vi "Configure-cameras.vi"(7 "Correct. params. ref.":refnum<data-value>, 8 "error in":errorcluster, 10 "Acquis. params. ref.":refnum<data-value>, 11 "Config. params. ref in.":refnum<data-value>) -> (0 "error IO":errorcluster, 3 "Config. params. ref.":refnum<data-value>, 5 "Succes?":bool)   [LabVIEW 2013, in "CameraVision.lvlib" / "CV-Configuration.lvclass"]
uses:
  CV-Configuration.lvclass
  Acquisition/CV-Acquisition.lvclass
  Correction/CV-Correction.lvclass
  Hardware/Camera/PF_MV1-D1312-240/PF_MV1-D1312-240.lvclass
  Hardware/Camera/Camera.lvclass
  UI/Module-states.ctl
  UI/Popup-messages.ctl
  Acquisition/CV-Acquisition.lvclass/CV-Acquisition.ctl
  CV-Configuration.lvclass/CV-Configuration.ctl
  Acquisition/Read Trigger mode.vi
  Acquisition/Read Maximum frame rate.vi
  Read Camport array.vi
  Read Framegrabber board.vi
  Read ROI width.vi
  Read ROI height.vi
  Read X-offsets.vi
  Read Y-offsets.vi
  Write Camera array.vi
  Write Camera status.vi
  UI/CV-UI.lvclass
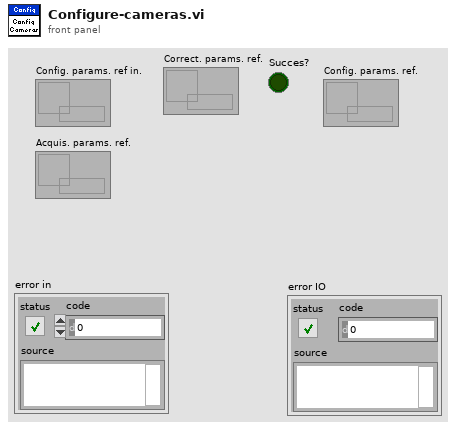
[diagram p1: front panel]
types:
  T1 = typedef "CameraVision.lvlib/CV-UI.lvclass/Popup-messages.ctl" = enum16{"Error-Black image", "Error-Camera config file", "Error-Camera connect", "Error-Grabber init", "Error-Camera setting", "Error-Image offset", "Error-Image import", "Error-Settings file not exist", "Error-Timing source", "Conflict-Filters", "Conflict-Map", "Conflict-Framerate", "Conflict-Charact", "Conflict-Temperature field", "Conflict-Temperature value", "Conflict-Storage-Binary image", "Conflict-Storage-Corrected image", "Conflict-Storage-Map", "Conflict-Storage-Charact", "Conflict-Storage-Temperature field", "Conflict-Storage-Temperature value", "Warning-File exist", "Warning-Parameter reset", "Warning-User cancel", "Info-Images imported"}
  T2 = typedef "CameraVision.lvlib/CV-UI.lvclass/Module-states.ctl" = enum16{"Inactive", "Active", "Data-loss", "Error", "Simulation", "Synchronizing", "Initialized", "Released"}
  T3 = typedef "Trigger-modes.ctl" = enum16{"Camera timed (not sync.)", "Framegrabber timed (sync.)", "Software timed (sync.)", "External timing (sync.)", "Manual (sync.)", "Gated - camera (not sync.)", "Gated - grabber (sync.)", "Gated - software (sync.)", "Gated - external (sync.)"}
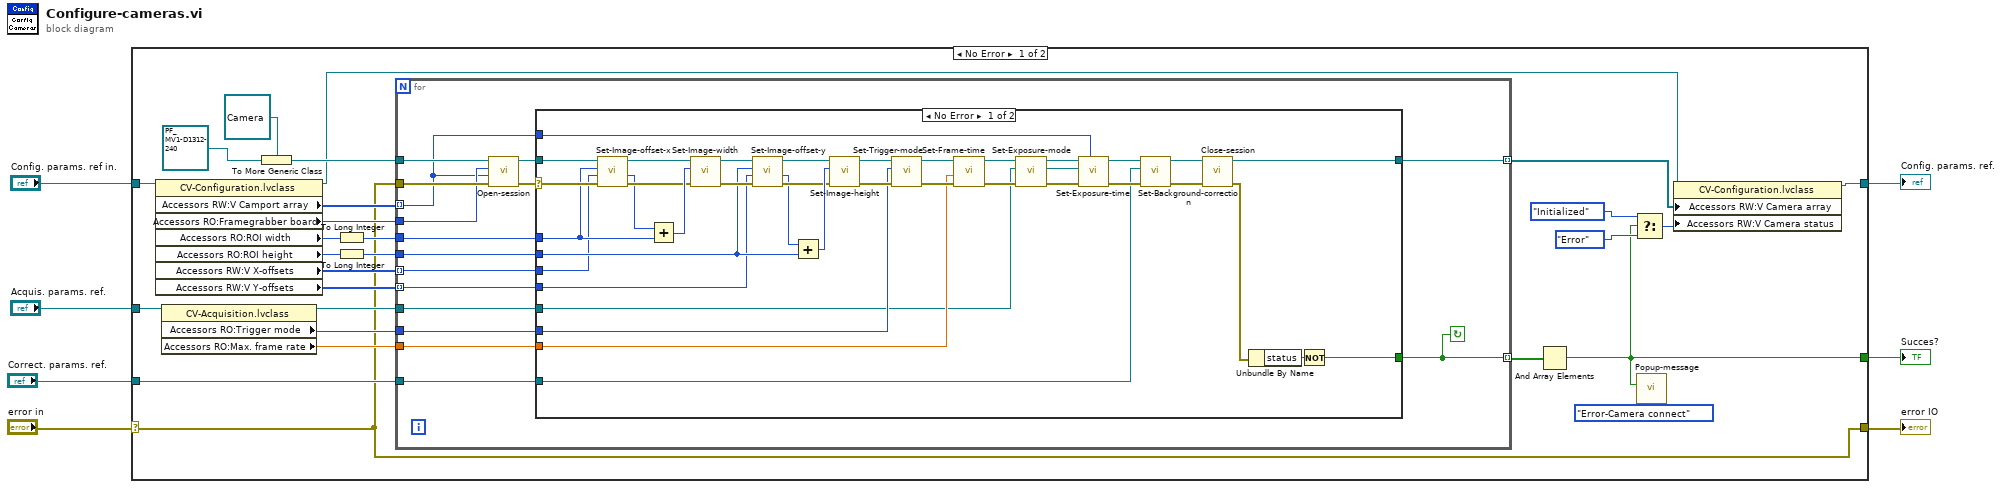
[diagram p0: block diagram]
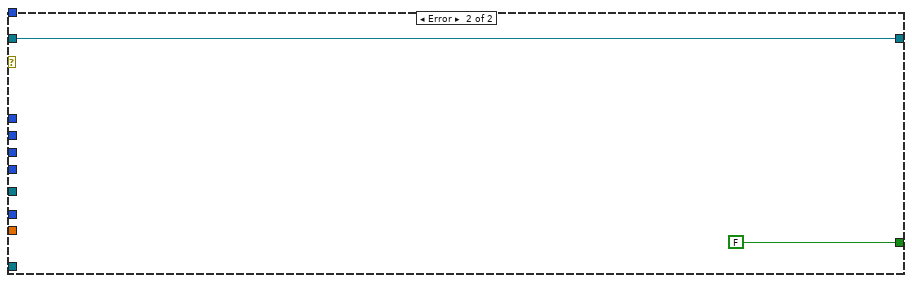
[diagram p2: hidden frame]
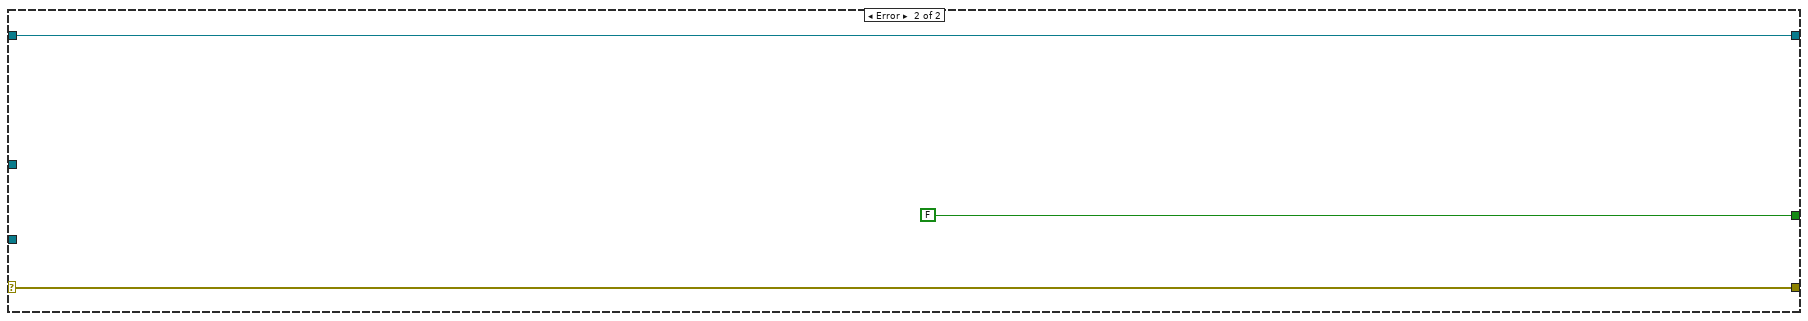
[diagram p3: hidden frame]
diagram:
  n1 = case shown="No Error" "error in" {
    selector: "error in" -> [w8 w93]
    tunnel: [w8 w93] -> w7
    tunnel: "Config. params. ref in." -> [w33 w91]
    tunnel: [w10 FALSE] -> w6
    tunnel: "Acquis. params. ref." -> [w32 _]
    tunnel: "Correct. params. ref." -> [w17 _]
    tunnel: [w22 w91] -> w1
    frame No Error {
      n2 = property class="CV-Configuration.lvclass"(reference=w33) -> (reference out=w23:refnum<data-value>, "Accessors RW:V Camport array"=w24:u32[], "Accessors RO:Framegrabber board"=w27:i32, "Accessors RO:ROI width"=w26:u32, "Accessors RO:ROI height"=w25:u32, "Accessors RW:V X-offsets"=w15:i32[], "Accessors RW:V Y-offsets"=w14:i32[])  [unwired: 1 in, 1 out]
      n3 = property class="CV-Acquisition.lvclass"(reference=w32) -> (reference out=w16:refnum<data-value>, "Accessors RO:Trigger mode"=w31:T3, "Accessors RO:Max. frame rate"=w18:dbl)  [unwired: 1 in, 1 out]
      n4 = To More Generic Class(target class=refnum<class "Camera.lvclass"> refnum ("Camera.lvclass"), reference=refnum<class "PF_MV1-D1312-240.lvclass"> refnum ("PF_MV1-D1312-240.lvclass")) -> (generic class reference=w28:refnum<class "Camera.lvclass">)
      n5 = To Long Integer(number=w26) -> (32bit integer=w20:i32)
      n6 = To Long Integer(number=w25) -> (32bit integer=w19:i32)
      n7 = for {
        tunnel: [w35] -> w34 mode=indexing
        tunnel: w20 -> [w50]
        tunnel: w19 -> [w49]
        tunnel: w31 -> [w48]
        tunnel: w18 -> [w47]
        tunnel: w8 -> [w46]
        tunnel: w28 -> [w43]
        tunnel: w24 -> [w36] mode=indexing
        tunnel: w27 -> [w42]
        tunnel: w15 -> [w40] mode=indexing
        tunnel: w14 -> [w41] mode=indexing
        tunnel: [w39] -> w21 mode=indexing
        tunnel: w17 -> [w38]
        tunnel: w16 -> [w37]
        stop <- w35 continue-if-true
        n8 = call-dynamic "Open-session.vi"("error in (no error)"=w46, "Camport"=w36, "Framegrabber board"=w42, "Camera in"=w43) -> ("error out"=w45:errorcluster, "Camera out"=w44:refnum<class "Camera.lvclass">)  [unwired: 5 in, 1 out]
        n9 = case shown="No Error" w45 {
          selector: w45 -> [w87 _]
          tunnel: w50 -> [w83 _]
          tunnel: [w60 FALSE] -> w35
          tunnel: w47 -> [w71 _]
          tunnel: w49 -> [w77 _]
          tunnel: w48 -> [w74 _]
          tunnel: w44 -> [w88 w90]
          tunnel: w41 -> [w58 _]
          tunnel: w40 -> [w59 _]
          tunnel: [w56 w90] -> w39
          tunnel: w38 -> [w53 _]
          tunnel: w37 -> [w52 _]
          tunnel: w36 -> [w57 _]
          frame No Error {
            n10 = call-dynamic "Set-Image-offset-x.vi"("error in (no error)"=w87, "Offset X in"=w59, "Image width"=w83, "Camera in"=w88) -> ("error out"=w85:errorcluster, "Offset X"=w62:i32, "Camera out"=w84:refnum<class "Camera.lvclass">)  [unwired: 5 in]
            n11 = Add(x=w62, y=w83) -> (x+y=w86:i32)
            n12 = call-dynamic "Set-Image-width.vi"("error in (no error)"=w85, "Image width in"=w86, "Camera in"=w84) -> ("error out"=w82:errorcluster, "Camera out"=w81:refnum<class "Camera.lvclass">)  [unwired: 5 in, 2 out]
            n13 = call-dynamic "Set-Image-offset-y.vi"("error in (no error)"=w82, "Offset Y in"=w58, "Image height"=w77, "Camera in"=w81) -> ("error out"=w79:errorcluster, "Offset Y"=w63:i32, "Camera out"=w78:refnum<class "Camera.lvclass">)  [unwired: 5 in]
            n14 = Add(x=w63, y=w77) -> (x+y=w80:i32)
            n15 = call-dynamic "Set-Image-height.vi"("error in (no error)"=w79, "Image height in"=w80, "Camera in"=w78) -> ("error out"=w75:errorcluster, "Camera out"=w76:refnum<class "Camera.lvclass">)  [unwired: 5 in, 2 out]
            n16 = call-dynamic "Set-Trigger-mode.vi"("error in (no error)"=w75, "Trigger mode"=w74, "Camera in"=w76) -> ("error out"=w73:errorcluster, "Camera out"=w72:refnum<class "Camera.lvclass">)  [unwired: 7 in]
            n17 = call-dynamic "Set-Frame-time.vi"("error in (no error)"=w73, "Frame rate"=w71, "Camera in"=w72) -> ("error out"=w69:errorcluster, "Camera out"=w70:refnum<class "Camera.lvclass">)  [unwired: 6 in, 1 out]
            n18 = call-dynamic "Set-Exposure-mode.vi"("error in (no error)"=w69, "Acquis. params. ref. in"=w52, "Camera in"=w70) -> ("error out"=w68:errorcluster, "Acquis. params. ref."=w51:refnum<data-value>, "Camera out"=w67:refnum<class "Camera.lvclass">)  [unwired: 6 in]
            n19 = call-dynamic "Set-Exposure-time.vi"("Camera"=w57, "error in (no error)"=w68, "Acquis. params. ref. in"=w51, "Camera in"=w67) -> ("error out"=w66:errorcluster, "Camera out"=w65:refnum<class "Camera.lvclass">)  [unwired: 4 in, 2 out]
            n20 = call-dynamic "Set-Background-correction.vi"("error in (no error)"=w66, "Correct. params in"=w53, "Camera in"=w65) -> ("error out"=w55:errorcluster, "Camera out"=w64:refnum<class "Camera.lvclass">)  [unwired: 6 in, 1 out]
            n21 = call-dynamic "Close-session.vi"("error in (no error)"=w55, "Camera in"=w64) -> ("error out"=w54:errorcluster, "Camera out"=w56:refnum<class "Camera.lvclass">)  [unwired: 6 in, 2 out]
            n22 = Unbundle By Name(w54) -> ("status"=w61:bool)
            n23 = Not(x=w61) -> (.not. x?=w60:bool)
          }
          frame Error {
          }
        }
      }
      n24 = And Array Elements(Boolean array=w34) -> (logical AND=w10:bool)
      n25 = Select(t=Module-states."Initialized" ("V Camera status"), s=w10, f=Module-states."Error" ("V Camera status")) -> (s? t:f=w11:T2)
      n26 = call "Popup-message.vi"("Message"=Popup-messages."Error-Camera connect", "Ignore?"=w10) -> ()  [unwired: 9 in, 1 out]
      n27 = property class="CV-Configuration.lvclass"(reference=w23, "Accessors RW:V Camera array"=w21, "Accessors RW:V Camera status"=w11) -> (reference out=w22:refnum<data-value>)  [unwired: 1 in, 1 out]
    }
    frame Error {
    }
  }
  "error IO" <- w7
  "Succes?" <- w6
  "Config. params. ref." <- w1
